vi "SCGlobVarsWrite.vi"(0 "dwellTime":u32=2000000, 1 "stop":bool, 2 "SPstate":T1, 3 "SPerrorCount":u8, 8 "writeStateOnly":bool, 9 "writeErrorCountOnly":bool) -> ()   [LabVIEW 2014]
uses:
  Controls/SPstate.ctl
  <vilib>/rvi/Emulation/niFpgaSctlEmulationGetInTimedLoop.vi
  SCGlobVars.vi
  <vilib>/rvi/Emulation/niFpgaProcessEmulError.vi
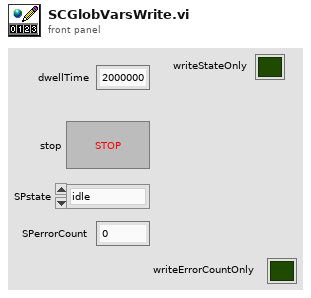
[diagram p1: front panel]
types:
  T1 = typedef "SPstate.ctl" = enum16{"idle", "scanning", "done", "error"}
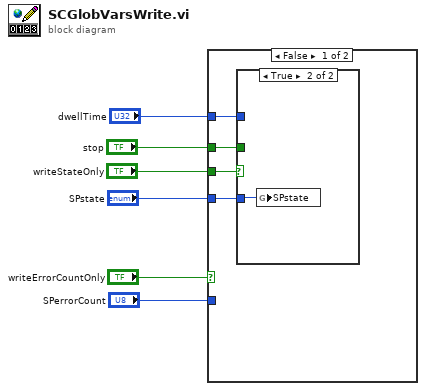
[diagram p0: block diagram]
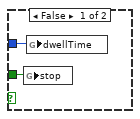
[diagram p2: hidden frame]
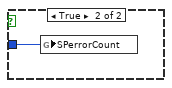
[diagram p3: hidden frame]
diagram:
  n1 = case shown="False" "writeErrorCountOnly" {
    tunnel: "writeStateOnly" -> [w10 _]
    tunnel: "SPstate" -> [w9 _]
    tunnel: "stop" -> [w8 _]
    tunnel: "dwellTime" -> [w7 _]
    tunnel: "SPerrorCount" -> [_ w14]
    frame False {
      n2 = case shown="True" w10 {
        tunnel: w9 -> [_ w13]
        tunnel: w8 -> [w12 _]
        tunnel: w7 -> [w11 _]
        frame False {
          n3 = global write "SCGlobVars.vi" "stop"(w12) -> ()
          n4 = global write "SCGlobVars.vi" "dwellTime"(w11) -> ()
        }
        frame True {
          n5 = global write "SCGlobVars.vi" "SPstate"(w13) -> ()
        }
      }
    }
    frame True {
      n6 = global write "SCGlobVars.vi" "SPerrorCount"(w14) -> ()
    }
  }
